vi "p2.vi"() -> ()   [LabVIEW 2025, in "d3.lvlib"]
uses:
  d3.lvlib
  lv2025-aoc/AOC/AOC.lvlib
  <userlib>/_OpenG.lib/string/string.llb/openg_string.lvlib
panel:
  in  "Example":string="987654321111111\n811111111111119\n234234234234278\n818181911112111"
  in  "Example 2":bool
  out "Answer":i64=7746
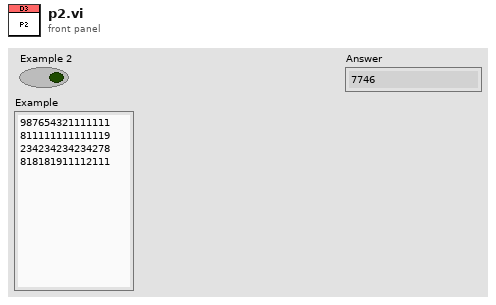
[diagram p1: front panel]
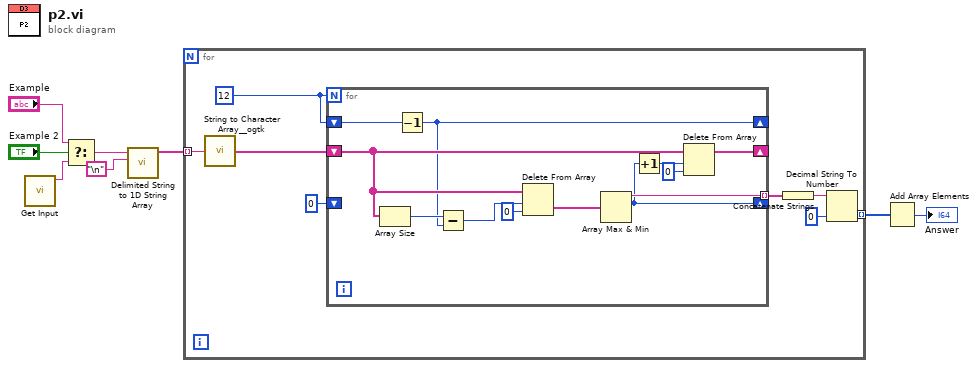
[diagram p0: block diagram]
diagram:
  n1 = call "Get Input.vi"() -> ("Input"=w8:string)  [unwired: 11 in]
  n2 = Select(t="Example", s="Example 2", f=w8) -> (s? t:f=w5:string)
  n3 = call <vilib>:"Delimited String to 1D String Array.vi"("delimiter"="\n", "delimited string"=w5) -> ("string array"=w3:string[])  [unwired: 9 in]
  n4 = for {
    tunnel: w3 -> [w16] mode=indexing
    tunnel: [w10] -> w1 mode=indexing
    w14 = 12
    n5 = call <userlib>:"String to Character Array__ogtk.vi"("Input String"=w16) -> ("Character Array"=w15:string[])
    n6 = for {
      N: w14 -> [_]
      shift-right: [w18] -> _
      shift-left: w14 -> [w22]
      tunnel: [w28] -> w12 mode=indexing
      shift-right: [w24] -> _
      shift-left: 0 -> [_]
      shift-right: [w26] -> _
      shift-left: w15 -> [w25]
      n7 = Array Size(array=w25) -> (size(s)=w27:i32)
      n8 = Decrement(x=w22) -> (x-1=w18:i32)
      n9 = Subtract(x=w27, y=w18) -> (x-y=w19:i32)
      n10 = Delete From Array(array=w25, length=w19, index=0) -> (deleted portion=w21:string[])  [unwired: 1 out]
      n11 = Array Max & Min(array=w21) -> (max value=w28:string, max index (indices)=w24:i32)  [unwired: 2 out]
      n12 = Increment(x=w24) -> (x+1=w17:i32)
      n13 = Delete From Array(array=w25, length=w17, index=0) -> (array with subset deleted=w26:string[])  [unwired: 1 out]
    }
    n14 = Concatenate Strings(w12) -> (w11:string)
    n15 = Decimal String To Number(string=w11, default (0L)=i64 0 ("default (0 I32)")) -> (number=w10:i64)  [unwired: 1 in, 1 out]
  }
  n16 = Add Array Elements(numeric array=w1) -> (sum=→"Answer":i64)
